vi "Shallow Copy and Deep Copy.vi"() -> ()   [LabVIEW 2017, in "Tree API.lvlib" / "Tree.lvclass"]
uses:
  Tree.lvclass
  API/Set Attribute Tree Data.vi
  Data Types/Int/To Integer Tree Data.vi
  Data Types/Int/Int.lvclass
  Data Types/String/To String Tree Data.vi
  Data Types/String/String.lvclass
  Data Types/Path/To Path Tree Data.vi
  Data Types/Path/Path.lvclass
panel:
  in  "Show IDs (True)":bool
  in  "After Deep Copy":string(tree)
  in  "After Shallow Copy":string(tree)
  in  "Before Copy":string(tree)
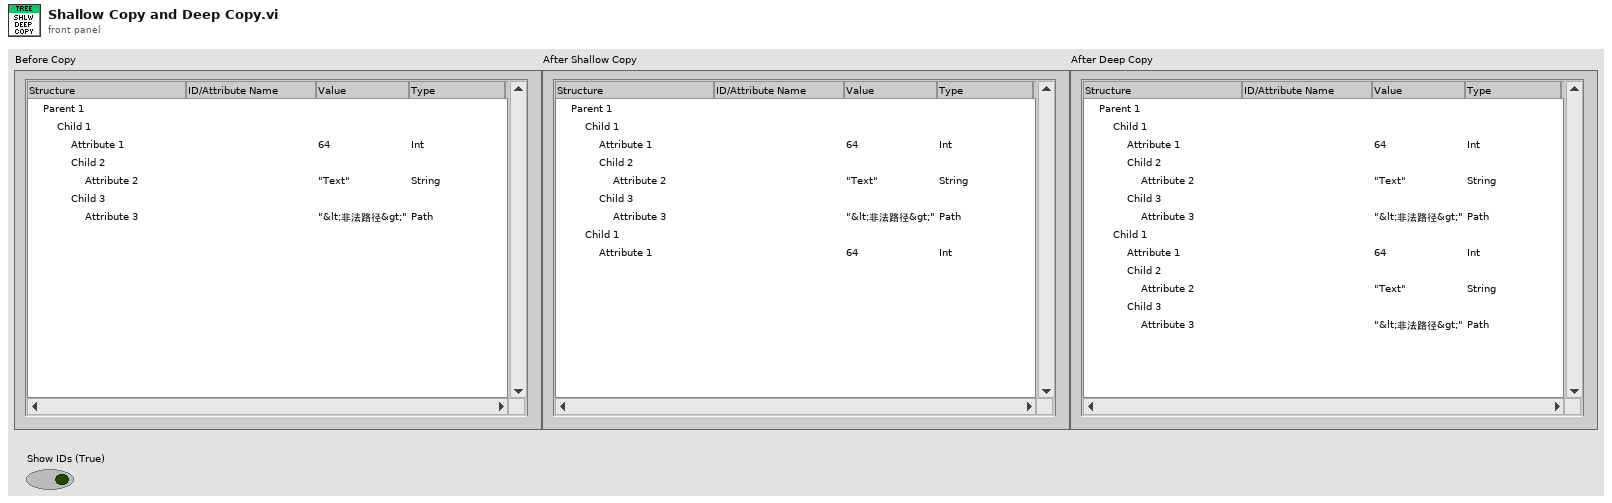
[diagram p1: front panel]
types:
  T1 = cluster{"Left Cell String":string, "Child Text":string[], "Child Tag":string, "Item Indent":i32, "Child Only?":bool, "Glyph Index":i32}[]
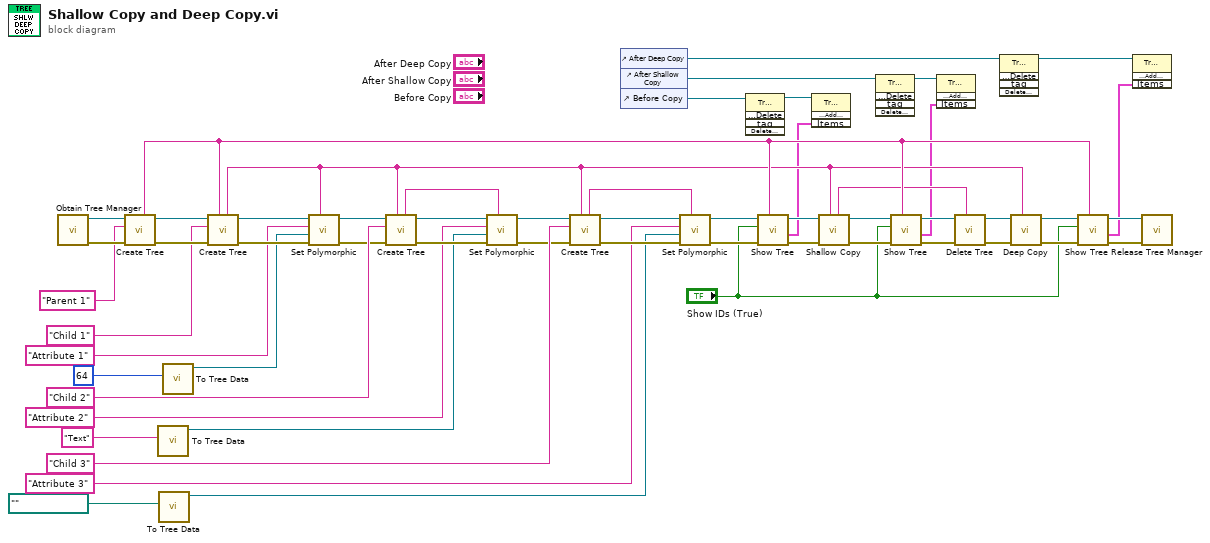
[diagram p0: block diagram]
diagram:
  n1 = call "Obtain Tree Manager.vi"() -> ("Error Out"=w55:errorcluster, "Tree"=w56:refnum<data-value>)  [unwired: 10 in]
  n2 = call "Create Tree.vi"("Error In"=w55, "Name"="Parent 1", "Tree Manager"=w56) -> ("Error Out"=w53:errorcluster, "Tree Manager"=w54:refnum<data-value>, "Unique ID"=w15:string)  [unwired: 6 in]
  n3 = call-poly "To Tree Data.vi"("String"="Text") -> ("String Tree Data"=w19:refnum<class "String.lvclass">)  [unwired: 10 in]
  n4 = call-poly "To Tree Data.vi"("Path"=path "" ("path")) -> ("Path Tree Data"=w17:refnum<class "Path.lvclass">)  [unwired: 10 in]
  n5 = call-poly "To Tree Data.vi"("Integer"=i64 64) -> ("Integer Tree Data"=w22:refnum<class "Int.lvclass">)  [unwired: 10 in]
  n6 = call "Create Tree.vi"("Parent ID (empty)"=w15, "Error In"=w53, "Name"="Child 1", "Tree Manager"=w54) -> ("Error Out"=w28:errorcluster, "Tree Manager"=w30:refnum<data-value>, "Unique ID"=w14:string)  [unwired: 5 in]
  n7 = call-poly "Set Polymorphic.vi"("Tree ID"=w14, "Error In"=w28, "Attribute Value"=w22, "Attribute Name"="Attribute 1", "Tree Manager"=w30) -> ("Error Out"=w27:errorcluster, "Tree Manager"=w29:refnum<data-value>)  [unwired: 4 in, 1 out]
  n8 = call "Create Tree.vi"("Parent ID (empty)"=w14, "Error In"=w27, "Name"="Child 2", "Tree Manager"=w29) -> ("Error Out"=w31:errorcluster, "Tree Manager"=w34:refnum<data-value>, "Unique ID"=w13:string)  [unwired: 5 in]
  n9 = call-poly "Set Polymorphic.vi"("Tree ID"=w13, "Error In"=w31, "Attribute Value"=w19, "Attribute Name"="Attribute 2", "Tree Manager"=w34) -> ("Error Out"=w32:errorcluster, "Tree Manager"=w33:refnum<data-value>)  [unwired: 4 in, 1 out]
  n10 = call "Create Tree.vi"("Parent ID (empty)"=w14, "Error In"=w32, "Name"="Child 3", "Tree Manager"=w33) -> ("Error Out"=w35:errorcluster, "Tree Manager"=w36:refnum<data-value>, "Unique ID"=w12:string)  [unwired: 5 in]
  n11 = control-ref of="After Deep Copy"() -> (w2:refnum<vi>)
  n12 = control-ref of="After Shallow Copy"() -> (w5:refnum<vi>)
  n13 = control-ref of="Before Copy"() -> (w8:refnum<vi>)
  n14 = call-poly "Set Polymorphic.vi"("Tree ID"=w12, "Error In"=w35, "Attribute Value"=w17, "Attribute Name"="Attribute 3", "Tree Manager"=w36) -> ("Error Out"=w25:errorcluster, "Tree Manager"=w26:refnum<data-value>)  [unwired: 4 in, 1 out]
  n15 = invoke class="Tree (严格)" method="Edit Tree Items.Delete"(reference=w8) -> (reference out=w10:refnum<vi>)  [unwired: 4 in, 4 out]
  n16 = call "Show Tree.vi"("Root ID"=w15, "Error In"=w25, "Show IDs (False)"="Show IDs (True)", "Tree"=w26) -> ("Error Out"=w47:errorcluster, "Items Out"=w7:T1, "Tree"=w48:refnum<data-value>)  [unwired: 5 in]
  n17 = invoke class="Tree (strict)" method="Edit Tree Items.Add Multiple Items to End"(reference=w10, "Items"=w7) -> ()  [unwired: 2 in, 4 out]
  n18 = call "Shallow Copy.vi"("Tree ID"=w14, "Error In"=w47, "Tree Manager"=w48) -> ("Error Out"=w45:errorcluster, "Tree Manager"=w46:refnum<data-value>, "Unique ID of Copied Tree"=w11:string)  [unwired: 6 in]
  n19 = invoke class="Tree (strict)" method="Edit Tree Items.Delete"(reference=w5) -> (reference out=w6:refnum<vi>)  [unwired: 4 in, 4 out]
  n20 = call "Show Tree.vi"("Root ID"=w15, "Error In"=w45, "Show IDs (False)"="Show IDs (True)", "Tree"=w46) -> ("Error Out"=w43:errorcluster, "Items Out"=w4:T1, "Tree"=w44:refnum<data-value>)  [unwired: 5 in]
  n21 = invoke class="Tree (strict)" method="Edit Tree Items.Add Multiple Items to End"(reference=w6, "Items"=w4) -> ()  [unwired: 2 in, 4 out]
  n22 = call "Delete Tree.vi"("Tree ID"=w11, "Error In"=w43, "Tree Manager"=w44) -> ("Error Out"=w41:errorcluster, "Tree Manager"=w42:refnum<data-value>)  [unwired: 7 in]
  n23 = invoke class="Tree (strict)" method="Edit Tree Items.Delete"(reference=w2) -> (reference out=w3:refnum<vi>)  [unwired: 4 in, 4 out]
  n24 = call "Deep Copy.vi"("Tree ID"=w14, "Error In"=w41, "Tree Manager"=w42) -> ("Error Out"=w39:errorcluster, "Tree Manager"=w40:refnum<data-value>)  [unwired: 6 in, 1 out]
  n25 = call "Show Tree.vi"("Root ID"=w15, "Error In"=w39, "Show IDs (False)"="Show IDs (True)", "Tree"=w40) -> ("Error Out"=w37:errorcluster, "Items Out"=w1:T1, "Tree"=w38:refnum<data-value>)  [unwired: 5 in]
  n26 = invoke class="Tree (strict)" method="Edit Tree Items.Add Multiple Items to End"(reference=w3, "Items"=w1) -> ()  [unwired: 2 in, 4 out]
  n27 = call "Release Tree Manager.vi"("Error In"=w37, "Tree"=w38) -> ()  [unwired: 9 in, 1 out]
